vi "3.2-Where.vi"() -> ()   [LabVIEW 2010]
uses:
  4-High Neurons/Current GPS Data.ctl
  3.2-Where/_typedefs/3.2.1-VectorNav Data.ctl
  3.0 Flow Control/3.0 List of Loops.ctl
  4-High Neurons/4.2-Where Sensor Typedef.ctl
  3.0-Global.vi
panel:
  out "Data":dbl[](array[numeric])
  out "4.2.1-VectorNav Status":string
  out "4.2.1-VectorNav Data":T1
  out "4.2.2-GPS Data":T2 {"Longitude (Decimal Degrees)" format="%#.6g"; "Lattitude (Decimal Degrees)" format="%#.6g"}
  # "GPS"
  # "VectorNav"
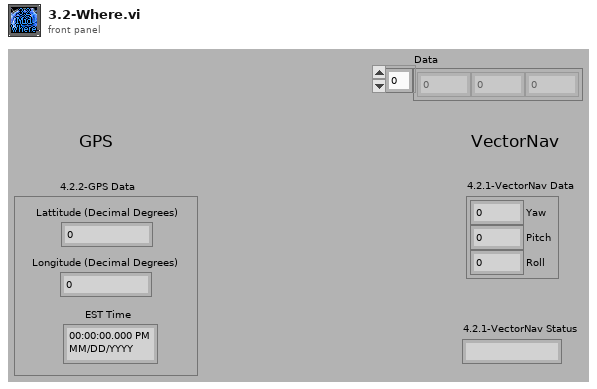
[diagram p1: front panel]
types:
  T1 = typedef "3.2.1-VectorNav Data.ctl" = cluster{"Yaw":dbl, "Pitch":dbl, "Roll":dbl}
  T2 = typedef "Current GPS Data.ctl" = cluster{"Lattitude (Decimal Degrees)":ext, "Longitude (Decimal Degrees)":ext, "EST Time":timestamp}
  T3 = typedef "3.0 List of Loops.ctl" = enum16{"3.0 State Update", "3.0 GUI", "3.1 Act", "3.1 4.7.1 Act UDP", "3.1 Joystick", "3.2 Where", "3.2 4.7.2 Where UDP", "3.3 What", "3.3 4.7.3 What UDP", "3.4 How", "3.4 4.7.4 How UDP", "3.5 Limbic", "3.8 TCP", "3.6 Cerebellum", "3.8 TCP Act"}
  T4 = typedef "4.2-Where Sensor Typedef.ctl" = cluster{"4.2.2- Current GPS Data":T2, "4.2.1-VectorNav Data":T1, "4.2.1-VectorNav Status":string}
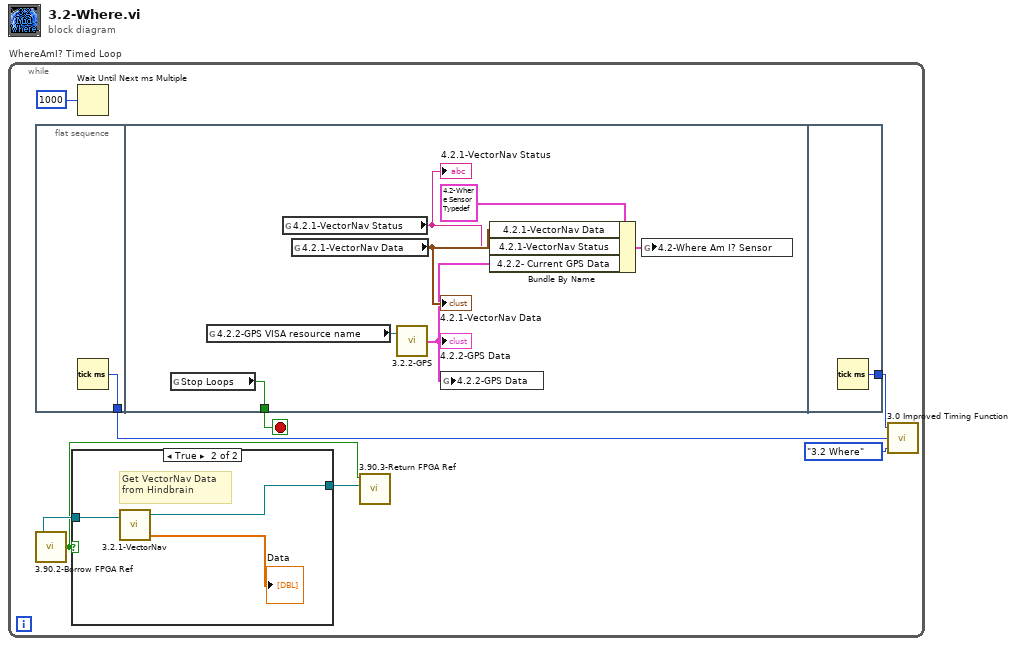
[diagram p0: block diagram]
diagram:
  n1 = while "WhereAmI? Timed Loop" {
    stop <- w8 stop-if-true
    n2 = flat-sequence {
      tunnel: [w13] -> w6
      tunnel: [w15] -> w8
      tunnel: [w21] -> w7
      frame #0 {
        n3 = Tick Count (ms)() -> (millisecond timer value=w13:u32)
      }
      frame #1 {
        n4 = global read "3.0-Global.vi" "Stop Loops"() -> (w15:bool)
        n5 = global read "3.0-Global.vi" "4.2.2-GPS VISA resource name"() -> (w14:refnum<visa-resource-name>)
        n6 = global read "3.0-Global.vi" "4.2.1-VectorNav Status"() -> (w18:string)
        "4.2.1-VectorNav Status" <- w18
        n7 = global read "3.0-Global.vi" "4.2.1-VectorNav Data"() -> (w19:T1)
        "4.2.1-VectorNav Data" <- w19
        n8 = call "3.2.2-GPS.vi"("VISA resource name"=w14) -> ("Current GPS Data"=w16:T2)  [unwired: 1 in]
        "4.2.2-GPS Data" <- w16
        n9 = global write "3.0-Global.vi" "4.2.2-GPS Data"(w16) -> ()
        n10 = Bundle By Name(cluster=T4 {"4.2.2- Current GPS Data"={"Lattitude (Decimal Degrees)"=0.0, "Longitude (Decimal Degrees)"=0.0, "EST Time"=timestamp(0 s since 1904-01-01)}, "4.2.1-VectorNav Data"={"Yaw"=0.0, "Pitch"=0.0, "Roll"=0.0}, "4.2.1-VectorNav Status"=""} ("Consolidated Where Data 2"), "4.2.1-VectorNav Data"=w19, "4.2.1-VectorNav Status"=w18, "4.2.2- Current GPS Data"=w16) -> (w17:T4)
        n11 = global write "3.0-Global.vi" "4.2-Where Am I? Sensor"(w17) -> ()
      }
      frame #2 {
        n12 = Tick Count (ms)() -> (millisecond timer value=w21:u32)
      }
    }
    n13 = call "3.90.2-Borrow FPGA Ref.vi"() -> ("Has Refrence"=w1:bool, "Ref Out"=w2:refnum<k20>)
    n14 = case shown="True" w1 {
      tunnel: [w9 w12] -> w3
      tunnel: w2 -> [w9 w11]
      frame False {
      }
      frame True {
        # "Get VectorNav Data from Hindbrain"
        n15 = call "3.2.1-VectorNav.vi"("FPGA Ref In"=w11) -> ("Data"=→"Data":dbl[], "FPGA Ref Out"=w12:refnum<k20>)  [unwired: 2 in]
      }
    }
    n16 = Wait Until Next ms Multiple(millisecond multiple=u32 1000) -> ()  [unwired: 1 out]
    n17 = call "3.90.3-Return FPGA Ref.vi"("element"=w3, "Has Refrence"=w1) -> ()  [unwired: 3 in]
    n18 = call "3.0 Improved Timing Function.vi"("Loop"=3.0_List_of_Loops."3.2 Where", "Start"=w6, "End"=w7) -> ()  [unwired: 1 in]
  }
